vi "SVL Limit Testing (XY).vi"(8 "error in (no error)":errorcluster, 9 "lower limit":cluster{"X":dbl[], "Y":dbl[]} {"X" format="%.2f"; "Y" format="%.2f"}, 10 "upper limit":cluster{"X":dbl[], "Y":dbl[]} {"X" format="%.2f"; "Y" format="%.2f"}, 11 "signal in":cluster{"X":dbl[], "Y":dbl[]} {"X" format="%.2f"; "Y" format="%.2f"}) -> (0 "error out":errorcluster, 1 "output values":cluster{"frequencies":dbl[], "spectrum":dbl[]}[](graph), 2 "test results":bool[](array[boolean]), 3 "test passed?":bool)   [LabVIEW 2017, in "SoundVib_LimitTest.lvlib"]
doc: "Performs limit testing on waveforms, spectra, XY data, identified peaks, or scalar measurements. You can specify an upper and lower boundary of the envelope to define a pass range. This VI uses the defined pass range to test the input signal. VI outputs apply only to the current input signal. You can wire output values to a graph to view the limits, signal, and failures. Wire data to the<B> signal in</B> input to determine the polymorphic instance to use or manually select the instance."
uses:
  <vilib>/addons/Sound and Vibration/svt_Limit Test/SoundVib_LimitTest.lvlib
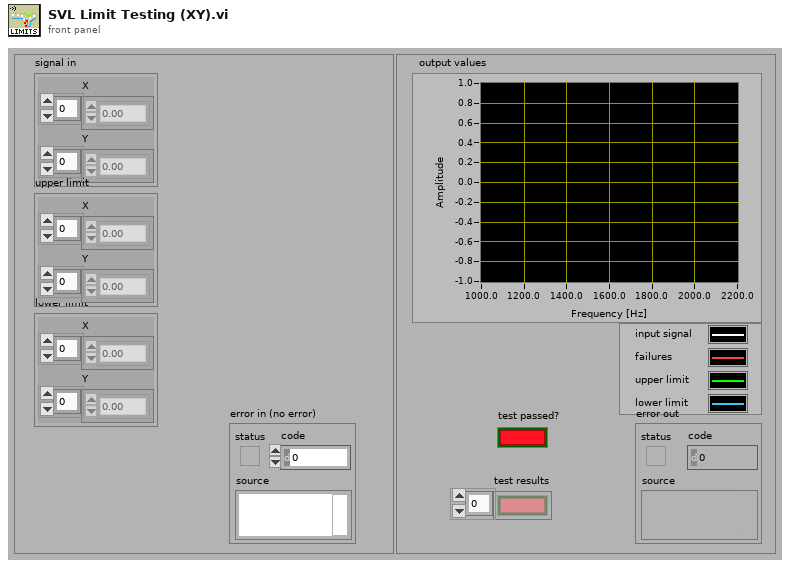
[diagram p1: front panel]
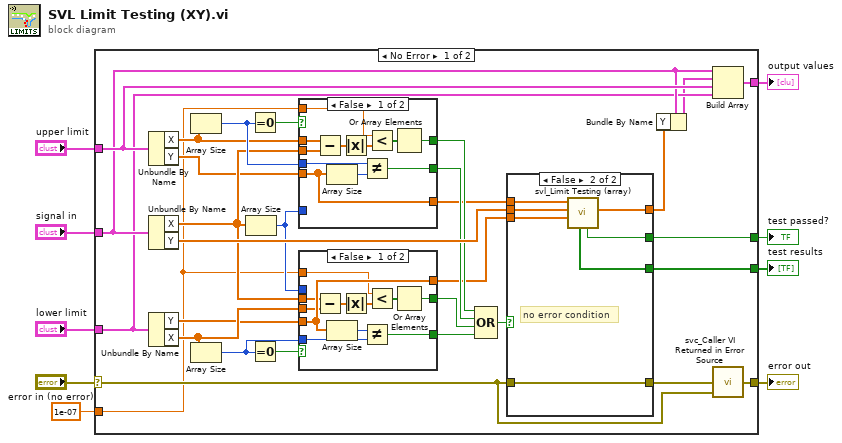
[diagram p0: block diagram]
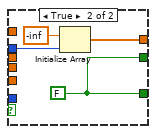
[diagram p2: hidden frame]
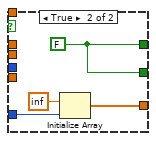
[diagram p3: hidden frame]
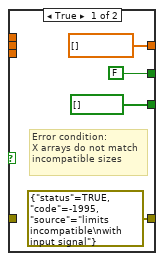
[diagram p4: hidden frame]
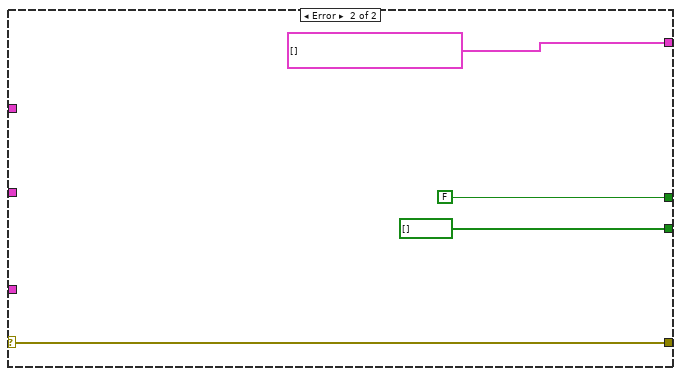
[diagram p5: hidden frame]
diagram:
  n1 = case shown="No Error" "error in (no error)" {
    selector: "error in (no error)" -> [w11 w84]
    tunnel: [w37 w84] -> w8
    tunnel: [w31 bool[] [] ("Array Constant")] -> w7
    tunnel: [w32 FALSE] -> w6
    tunnel: "upper limit" -> [w36 _]
    tunnel: "signal in" -> [w35 _]
    tunnel: "lower limit" -> [w30 _]
    tunnel: [w34 cluster{"X":dbl[], "Y":dbl[]}[] []] -> w2
    tunnel: 1e-07 -> [w10 _]
    frame No Error {
      n2 = Unbundle By Name(w36) -> ("X"=w33:dbl[], "Y"=w16:dbl[])
      n3 = Unbundle By Name(w35) -> ("X"=w17:dbl[], "Y"=w27:dbl[])
      n4 = Unbundle By Name(w30) -> ("Y"=w15:dbl[], "X"=w23:dbl[])
      n5 = Array Size(array=w33) -> (size(s)=w39:i32)
      n6 = Array Size(array=w23) -> (size(s)=w24:i32)
      n7 = Array Size(array=w17) -> (size(s)=w14:i32)
      n8 = Equal To 0?(x=w39) -> (x = 0?=w25:bool)
      n9 = Equal To 0?(x=w24) -> (x = 0?=w22:bool)
      n10 = case shown="False" w25 {
        tunnel: w17 -> [w64 _]
        tunnel: w39 -> [w63 _]
        tunnel: w33 -> [w62 _]
        tunnel: [w61 w69] -> w20
        tunnel: [w56 w69] -> w21
        tunnel: w16 -> [w60 _]
        tunnel: w14 -> [_ w68]
        tunnel: [w60 w66] -> w13
        tunnel: w10 -> [w58 _]
        frame False {
          n11 = Subtract(x=w62, y=w64) -> (x-y=w59:dbl[])
          n12 = Array Size(array=w60) -> (size(s)=w65:i32)
          n13 = Absolute Value(x=w59) -> (abs(x)=w55:dbl[])
          n14 = Not Equal?(x=w63, y=w65) -> (x != y?=w61:bool)
          n15 = Less?(x=w58, y=w55) -> (x < y?=w57:bool[])
          n16 = Or Array Elements(Boolean array=w57) -> (logical OR=w56:bool)
        }
        frame True {
          w69 = FALSE
          n17 = Initialize Array(inf ("element"), w68) -> (w66:dbl[])
        }
      }
      n18 = case shown="False" w22 {
        tunnel: w23 -> [w43 _]
        tunnel: w24 -> [w48 _]
        tunnel: w17 -> [w44 _]
        tunnel: [w50 w54] -> w18
        tunnel: [w42 w54] -> w19
        tunnel: w15 -> [w47 _]
        tunnel: w14 -> [_ w53]
        tunnel: [w47 w51] -> w12
        tunnel: w10 -> [w41 _]
        frame False {
          n19 = Subtract(x=w44, y=w43) -> (x-y=w46:dbl[])
          n20 = Array Size(array=w47) -> (size(s)=w49:i32)
          n21 = Absolute Value(x=w46) -> (abs(x)=w40:dbl[])
          n22 = Not Equal?(x=w49, y=w48) -> (x != y?=w50:bool)
          n23 = Less?(x=w41, y=w40) -> (x < y?=w45:bool[])
          n24 = Or Array Elements(Boolean array=w45) -> (logical OR=w42:bool)
        }
        frame True {
          w54 = FALSE
          n25 = Initialize Array(-inf ("element"), w53) -> (w51:dbl[])
        }
      }
      n26 = Compound Arithmetic op=OR(w21, w20, w19, w18) -> (w28:bool)
      n27 = case shown="False" w28 {
        tunnel: w11 -> [_ w80]
        tunnel: [errorcluster {"status"=TRUE, "code"=-1995, "source"="limits incompatible\nwith input signal"} ("error IO") w80] -> w38
        tunnel: [dbl[] [] ("failure array") w74] -> w26
        tunnel: [FALSE ("test passed") w76] -> w32
        tunnel: [bool[] [] ("test results") w75] -> w31
        tunnel: w13 -> [_ w79]
        tunnel: w27 -> [_ w78]
        tunnel: w12 -> [_ w77]
        frame True {
          # "Error condition:\nX arrays do not match\nincompatible sizes"
        }
        frame False {
          # "no error condition"
          n28 = call <vilib>:"svl_Limit Testing (array).vi"("lower limit"=w77, "input array"=w78, "upper limit"=w79) -> ("failure array"=w74:dbl[], "test passed"=w76:bool, "test results"=w75:bool[])  [unwired: 4 in, 2 out]
        }
      }
      n29 = Bundle By Name(cluster=w35, "Y"=w26) -> (w29:cluster{"X":dbl[], "Y":dbl[]})
      n30 = Build Array(w35, w29, w36, w30) -> (w34:cluster{"X":dbl[], "Y":dbl[]}[])
      n31 = call <vilib>:"svc_Caller VI Returned in Error Source.vi"("warning input to caller"=w11, "error in (no error)"=w38) -> ("error out"=w37:errorcluster)  [unwired: 3 in]
    }
    frame Error {
    }
  }
  "error out" <- w8
  "output values" <- w2
  "test passed?" <- w6
  "test results" <- w7
